vi "Get 4 Tables BY RH.vi"(0 "Air Pressure [psia]":dbl, 3 "Relative Humidity [%]":dbl) -> (1 "Pressure Z":dbl, 4 "RH Z":dbl, 5 "HP Higher RH Psych Table":dbl[][](array[numeric]), 6 "HP Lower RH Psych Table":dbl[][](array[numeric]), 7 "LP Higher RH Psych Table":dbl[][](array[numeric]), 8 "LP Lower RH Psych Table":dbl[][](array[numeric]))   [LabVIEW 2020]
panel:
  in  "RH Array":dbl[](array[numeric])=[0.0, 10.0, 20.0, 30.0, 40.0, 50.0, 60.0, 70.0, 80.0, 90.0, 100.0]
  in  "Pressure Array":dbl[](array[numeric])=[15.51026974, 15.23488864, 14.96348006, 14.696, 14.43240481, 14.17265118, 13.91669613, 13.66449702, 13.41601153, 13.17119769, 12.93001384, 12.69241866, 12.45837117, 12.22783068, 12.00075687, 11.77710969, 11.55684946, 11.3399368]
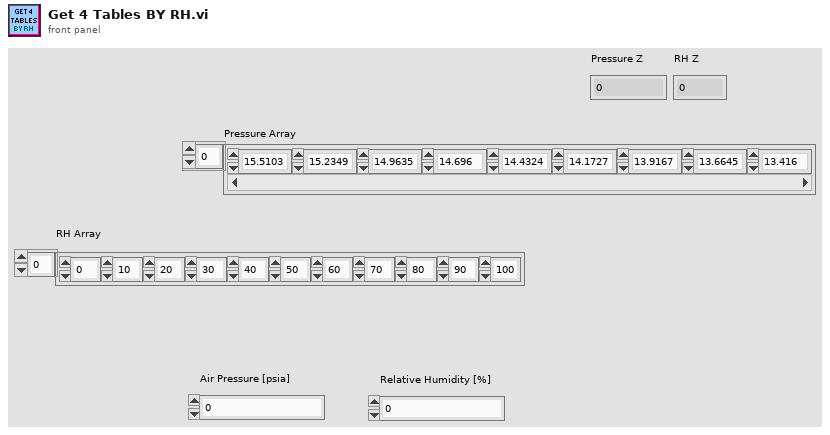
[diagram p1: front panel]
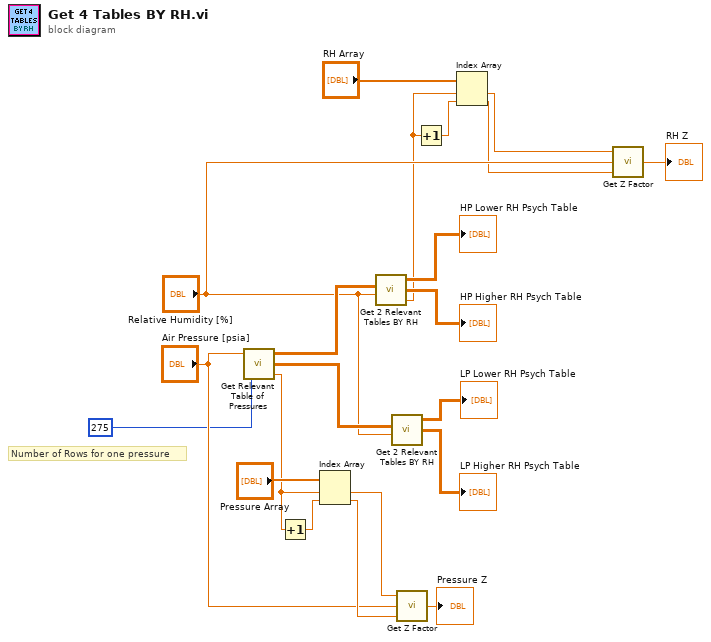
[diagram p0: block diagram]
diagram:
  # "Number of Rows for one pressure"
  n1 = call "Get Relevant Table of Pressures.vi"("Length of List for 1 Pressure"=275 ("Length of List for a Single Pressure"), "Air Pressure [psia]"="Air Pressure [psia]") -> ("Pressure Index"=w12:dbl, "Lower Pressure Psych Table"=w18:dbl[][], "Higher Pressure Psych Table"=w21:dbl[][])  [unwired: 1 in]
  n2 = Increment(x=w12) -> (x+1=w11:dbl)
  n3 = Index Array(array="Pressure Array", index #1=w12, index #2=w11) -> (element #1=w10:dbl, element #2=w9:dbl)
  n4 = call "Get 2 Relevant Tables BY RH.vi"("Psych Table"=w21, "Relative Humidity"="Relative Humidity [%]") -> ("Lower RH Psych Table"=→"HP Lower RH Psych Table":dbl[][], "Higher RH Psych Table"=→"HP Higher RH Psych Table":dbl[][], "RH Index"=w6:dbl)  [unwired: 4 in]
  n5 = call "Get 2 Relevant Tables BY RH.vi"("Psych Table"=w18, "Relative Humidity"="Relative Humidity [%]") -> ("Lower RH Psych Table"=→"LP Lower RH Psych Table":dbl[][], "Higher RH Psych Table"=→"LP Higher RH Psych Table":dbl[][])  [unwired: 4 in, 1 out]
  n6 = call "Get Z Factor.vi"("X2"=w9, "Xi"="Air Pressure [psia]", "X1"=w10) -> ("Z"=→"Pressure Z":dbl)  [unwired: 2 in]
  n7 = Increment(x=w6) -> (x+1=w7:dbl)
  n8 = Index Array(array="RH Array", index #1=w6, index #2=w7) -> (element #1=w5:dbl, element #2=w4:dbl)
  n9 = call "Get Z Factor.vi"("X2"=w4, "Xi"="Relative Humidity [%]", "X1"=w5) -> ("Z"=→"RH Z":dbl)  [unwired: 2 in]
